vi "Plugin.UDP.Get Custom Properties (single).vi"(10 "id":i32, 11 "UDP Plugin in":refnum<class "UDP Plugin.lvclass">) -> (2 "custom properties":cluster{"port":u16}, 3 "UDP Plugin out":refnum<class "UDP Plugin.lvclass">)   [LabVIEW 2016, in "UDP Plugin.lvclass"]
uses:
  UDP Plugin.lvclass
  UDP Plugin.lvclass/UDP Plugin.ctl
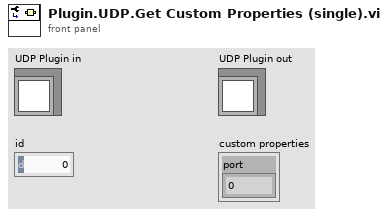
[diagram p1: front panel]
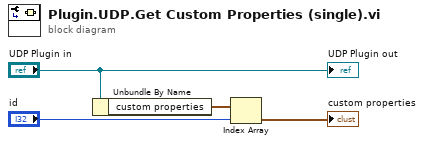
[diagram p0: block diagram]
diagram:
  n1 = Unbundle By Name("UDP Plugin in") -> ("custom properties"=w3:cluster{"port":u16}[])
  n2 = Index Array(array=w3, index="id") -> (element=→"custom properties":cluster{"port":u16})
  "UDP Plugin out" <- "UDP Plugin in"
